vi "Set Iteration Count.vi"(8 "error in (no error)":errorcluster, 11 "For Loop Dialog in":refnum<class "Name Only Dialog.lvclass">) -> (0 "error out":errorcluster, 3 "For Loop Dialog out":refnum<class "Name Only Dialog.lvclass">)   [LabVIEW 2017]
uses:
  ITest Executive Builder Dialog/ITest Executive Builder Dialog.lvclass
  Name Only Dialog.lvclass
  C:/Users/jonmc/Documents/Git/Test Executive Builder/Source/Test Executive Builder Dialogs/ITest Executive Builder Dialog/ITest Executive Builder Dialog.lvclass
  C:/Users/jonmc/Documents/Git/Test Executive Builder/gpm_packages/@cs/mva-framework/Source/Framework/IDialogBox/IDialogBox/IDialogBox.lvclass
  C:/Users/jonmc/Documents/Git/Test Executive Builder/gpm_packages/@cs/mva-framework/Source/Framework/IViewable/IViewable/IViewable.lvclass
  C:/Users/jonmc/Documents/Git/Test Executive Builder/gpm_packages/@cs/mva-framework/Source/Framework/ActorEvents/IEventAggregator/IEventAggregator.lvclass
  C:/Users/jonmc/Documents/Git/Test Executive Builder/gpm_packages/@cs/mva-framework/Source/Framework/IObserver/IObserver/IObserver.lvclass
  C:/Program Files (x86)/National Instruments/LabVIEW 2017/vi.lib/ActorFramework/Actor/Actor.lvclass
  gpm_packages/@cs/test-executive/Source/Test Executive/TestExecutive Ref/TestExecutive Ref.lvclass
  dd497790-5a6f-4032-9eef-5518b3fbc898.vi
  98711db4-5abe-4e61-829e-3a8c06daad23.vi
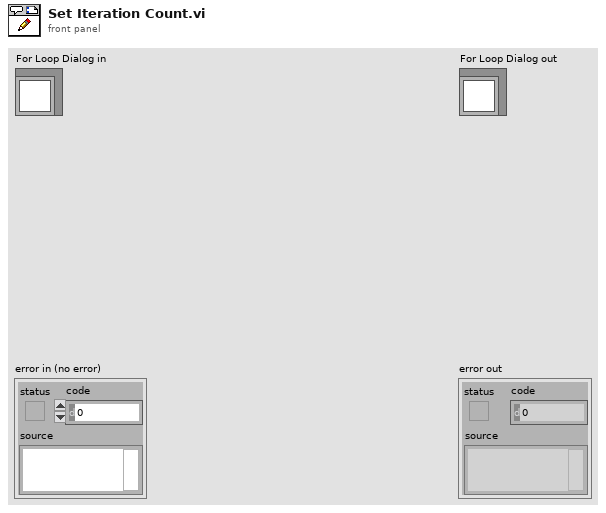
[diagram p1: front panel]
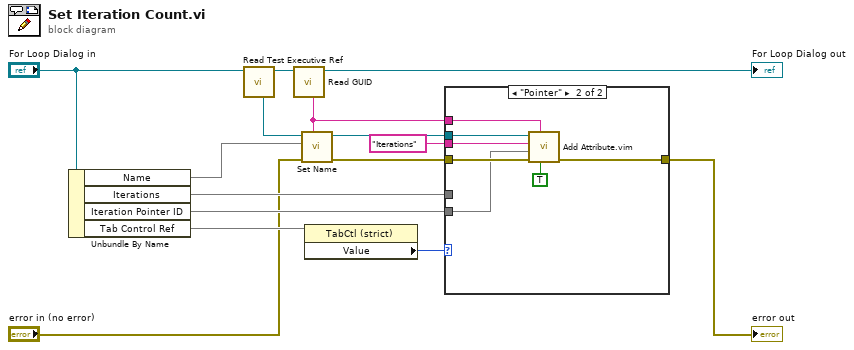
[diagram p0: block diagram]
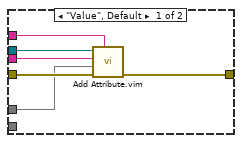
[diagram p2: hidden frame]
diagram:
  n1 = Unbundle By Name("For Loop Dialog in") -> ("Name"=w11, "Iterations"=w8, "Iteration Pointer ID"=w7, "Tab Control Ref"=w10)
  n2 = call "Read Test Executive Ref.vi"("ITest Executive Builder Dialog in"="For Loop Dialog in") -> ("ITest Executive Builder Dialog out"=w15:refnum<class "Name Only Dialog.lvclass">, "Test Executive Ref"=w12:refnum<data-value>)  [unwired: 9 in]
  n3 = call "Read GUID.vi"("ITest Executive Builder Dialog in"=w15) -> ("ITest Executive Builder Dialog out"=→"For Loop Dialog out":refnum<class "Name Only Dialog.lvclass">, "GUID"=w5:string)  [unwired: 9 in]
  n4 = call "Set Name.vi"("Unique ID"=w5, "error in (no error)"="error in (no error)", "Name"=w11, "Test Executive Ref"=w12) -> ("error out"=w3:errorcluster, "Test Executive Ref out"=w6:refnum<data-value>)  [unwired: 6 in]
  n5 = property class="TabCtl (strict)"(reference=w10) -> ("Value"=w9:enum32{"Value", "Pointer"})  [unwired: 1 in, 2 out]
  n6 = case shown="\"Pointer\"" w9 {
    tunnel: w8 -> [w17 _]
    tunnel: w7 -> [_ w24]
    tunnel: w6 -> [w21 w28]
    tunnel: w5 -> [w20 w23]
    tunnel: "Iterations" -> [w19 w25]
    tunnel: w3 -> [w18 w27]
    tunnel: [w16 w22] -> w1
    frame "Value", Default {
      n7 = call "Add Attribute.vim"("ID"=w20, "error in (no error)"=w18, "Attribute"=w17, "Attribute Name"=w19, "Test Executive Ref"=w21) -> ("error out"=w16:errorcluster)  [unwired: 3 in, 3 out]
    }
    frame "Pointer" {
      n8 = call "Add Attribute.vim"("Pointer?"=TRUE, "ID"=w23, "error in (no error)"=w27, "Attribute"=w24, "Attribute Name"=w25, "Test Executive Ref"=w28) -> ("error out"=w22:errorcluster)  [unwired: 2 in, 3 out]
    }
  }
  "error out" <- w1
